vi "Cryostat JSON.vi"(10 "<JSON>":string="{\"Target Field (T)\":0,\"Target Rate (T/min)\":0,\"Axis\":\"Z\",\"Mode\":\"Persistent\"}", 11 "Instrument.Cryostat in":refnum<class "Instrument.Cryostat.lvclass">) -> ()   [LabVIEW 2019, in "Instrument.Cryostat.lvclass"]
uses:
  Instrument.Cryostat.lvclass
  Typedefs/Magnet Mode--Enum.ctl
  Typedefs/Magnet Axis--Enum.ctl
  6d71229b-81e7-4ab7-93e2-5ff89073f8dd.vi
  57534547-750b-436d-a0c5-4d9fe28caa50.vi
  1822db08-b1c5-45d0-8edc-53e3a80cee39.vi
  e61b0bf3-2057-4b3d-882e-a9f6f05384d9.vi
  62ec00bf-e8a0-43ec-a3db-990e649f62d4.vi
  <vilib>/JDP Science/JSONtext/Find Item.vi
  <vilib>/JDP Science/JSONtext/String Subset.vi
  <vilib>/JDP Science/JSONtext/JSON text to Variant.vi
  <vilib>/JDP Science/JSONtext/Variant to JSON Text.vi
  <vilib>/JDP Science/JSONtext/Parsing/Parse Full Path or Item Name.vi
  <vilib>/JDP Science/JSONtext/Next JSON Value.vi
  <vilib>/JDP Science/JSONtext/support/Error Cluster From Code.vi
  <vilib>/JDP Science/JSONtext/Offset/Find Item Locations by Path.vi
  <vilib>/JDP Science/JSONtext/LVClass Serializer/JSONtext LVClass Serializer.lvclass
panel:
  out "Data":dbl
  out "error out":errorcluster
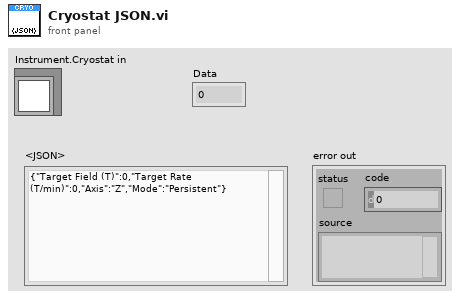
[diagram p1: front panel]
types:
  T1 = typedef "Instrument.Cryostat.lvclass/Magnet Axis--Enum.ctl" = enum16{"Z", "X", "Y"}
  T2 = typedef "Instrument.Cryostat.lvclass/Magnet Mode--Enum.ctl" = enum16{"Persistent", "Driven"}
  T3 = cluster{"Target Field (T)":dbl, "Target Rate (T/min)":dbl, "Axis":T1, "Mode":T2}
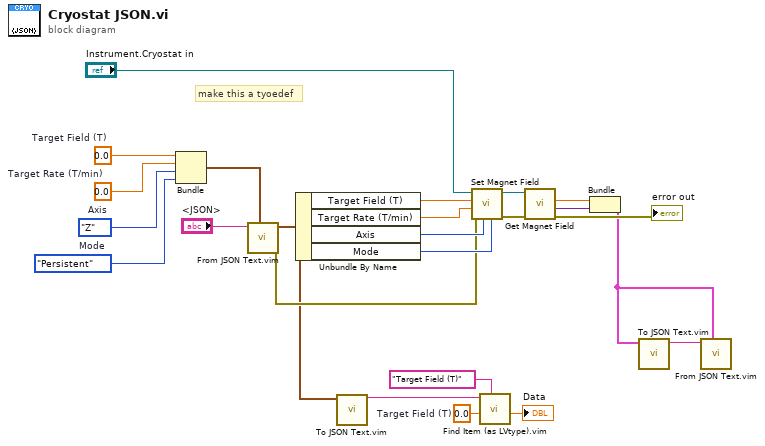
[diagram p0: block diagram]
diagram:
  w5 = 0.0  # Target Field (T)
  w12 = 0.0  # Target Field (T)
  w11 = 0.0  # Target Rate (T/min)
  w1 = Magnet_Axis--Enum."Z"  # Axis
  w2 = Magnet_Mode--Enum."Persistent"  # Mode
  # "make this a tyoedef"
  n1 = Bundle("Target Field (T)"=w12, "Target Rate (T/min)"=w11, "Axis"=w1, "Mode"=w2) -> (w20:T3)  [unwired: 1 in]
  n2 = call "From JSON Text.vim"("Data Type and Default Value"=w20, "JSON"="<JSON>") -> ("error out"=w15:errorcluster, "Data out"=w3:T3)  [unwired: 8 in]
  n3 = Unbundle By Name(w3) -> ("Target Field (T)"=w19:dbl, "Target Rate (T/min)"=w18:dbl, "Axis"=w17:T1, "Mode"=w16:T2)
  n4 = call "To JSON Text.vim"("Anything"=w3) -> ("<JSON>"=w7:string)  [unwired: 9 in, 1 out]
  n5 = call-dynamic "Set Magnet Field.vi"("Mode"=w16, "Axis"=w17, "error in (no error)"=w15, "Target Rate (T/min)"=w18, "Target Field (T)"=w19, "Instrument.Cryostat in"="Instrument.Cryostat in") -> ("error out"=w10:errorcluster, "Instrument.Cryostat out"=w13:refnum<class "Instrument.Cryostat.lvclass">)  [unwired: 4 in]
  n6 = call "Find Item (as LVtype).vim"("$Path or Item Name"="Target Field (T)", "Data Type and Default Value"=w5, "JSON"=w7) -> ("Data"=→"Data":dbl)  [unwired: 5 in, 3 out]
  n7 = call-dynamic "Get Magnet Field.vi"("error in (no error)"=w10, "Instrument.Cryostat in"=w13) -> ("error out"=→"error out":errorcluster, "Status"=w23:variant, "B Field (T)"=w24:dbl)  [unwired: 5 in, 2 out]
  n8 = Bundle("B Field (T)"=w24, "Status"=w23) -> (w8:cluster{"B Field (T)":dbl, "Status":variant})  [unwired: 1 in]
  n9 = call "To JSON Text.vim"("Anything"=w8) -> ("<JSON>"=w9:string)  [unwired: 9 in, 1 out]
  n10 = call "From JSON Text.vim"("Data Type and Default Value"=w8, "JSON"=w9) -> ()  [unwired: 8 in, 2 out]
